vi "Add Namer With Folder.vi"   [LabVIEW 2020, in "Approval Tests.lvlib"]
doc: "Drops everything needed to put approve and recieved files in a subfolder."
uses:
  Approval Tests.lvlib
  Options/Options.lvclass
  Namer with Folder/Namer with Folder.lvclass
  Options/Write Namer.vi
  C:/Users/SAS/Desktop/ApprovalTests.LabVIEW/Source/Approval Tests/Namer/Namer.lvclass
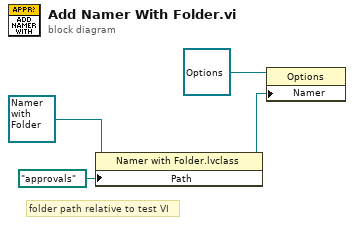
[diagram p0: block diagram]
diagram:
  # "folder path relative to test VI"
  n1 = property class="Namer with Folder.lvclass"(reference=refnum<class "Namer with Folder.lvclass"> refnum ("Approval Tests.lvlib:Regex Scrubber"), "Path"=path "approvals") -> (reference out=w2:refnum<class "Namer with Folder.lvclass">)  [unwired: 1 in, 1 out]
  n2 = property class="Options"(reference=refnum<class "Options.lvclass"> refnum ("Approval Tests.lvlib:Options"), "Namer"=w2) -> ()  [unwired: 1 in, 2 out]
